vi "Lex String.vi"(8 "error in (no error)":errorcluster, 11 "JSON Lexer in":refnum<class "JSON Lexer.lvclass">) -> (0 "error out":errorcluster, 1 "EOF":bool, 2 "Next State":T1=enum."Value", 3 "JSON Lexer out":refnum<class "JSON Lexer.lvclass">)   [LabVIEW 2013, in "JKI JSON Serialization.lvlib" / "JSON Lexer.lvclass"]
uses:
  JSON Lexer.lvclass
  JSON Lexer States.ctl
  JSON Lexer.lvclass/JSON Lexer.ctl
  <vilib>/addons/_JKI.lib/Unicode/UTF-8 String/UTF-8 String.lvclass/UTF-8 String.ctl
  JSON Token Type.ctl
  <vilib>/addons/_JKI.lib/Unicode/UTF-8 String/Index Rune as UTF-8 Substring.vi
  <vilib>/addons/_JKI.lib/Unicode/UTF-8 String/Next Rune As UTF-8 Substring.vi
  <vilib>/addons/_JKI.lib/Unicode/UTF-8 String/Bytes In Rune.vi
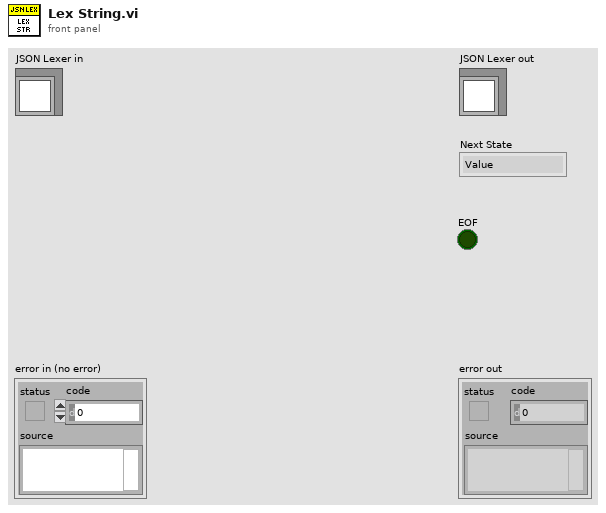
[diagram p1: front panel]
types:
  T1 = typedef "JKI JSON Serialization.lvlib/JSON Lexer.lvclass/JSON Lexer States.ctl" = enum16{"Undefined", "Value", "String", "Numeric", "Number", "Symbol", "Symbolic Number"}
  T2 = typedef "JKI JSON Serialization.lvlib/JSON Lexer.lvclass/JSON Token Type.ctl" = enum32{"unknown", "comma", "end-label", "begin-object", "end-object", "begin-array", "end-array", "quoted-string", "boolean", "exponential-number", "decimal-number", "integer-number", "special-number", "null", "symbol", "whitespace", "EOF"}
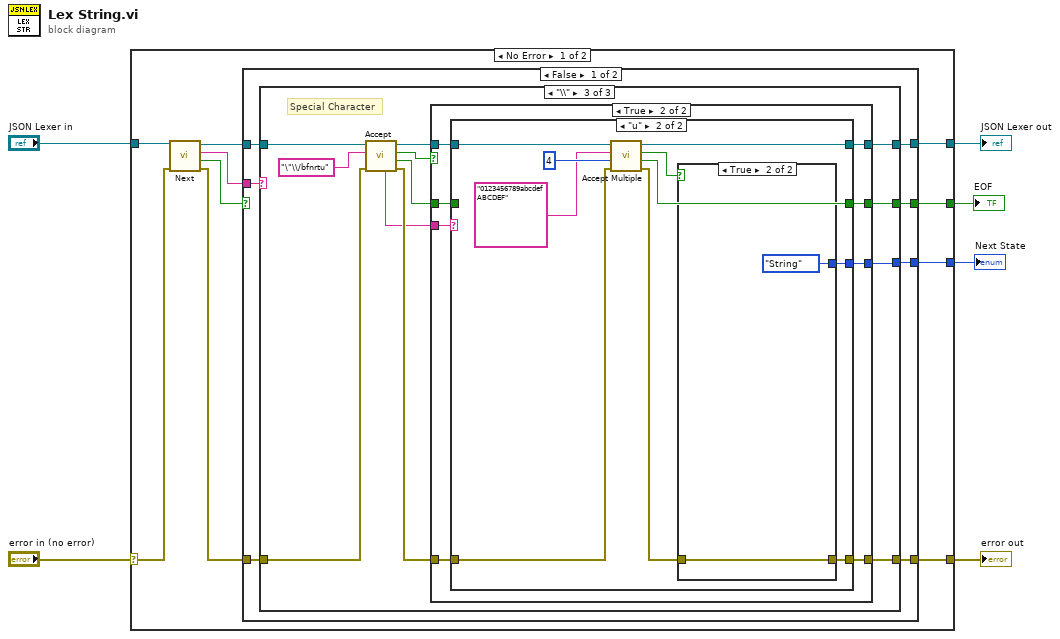
[diagram p0: block diagram]
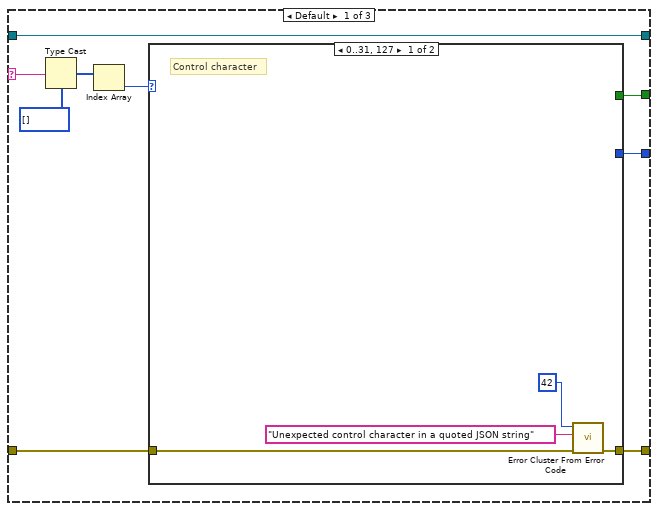
[diagram p2: hidden frame]
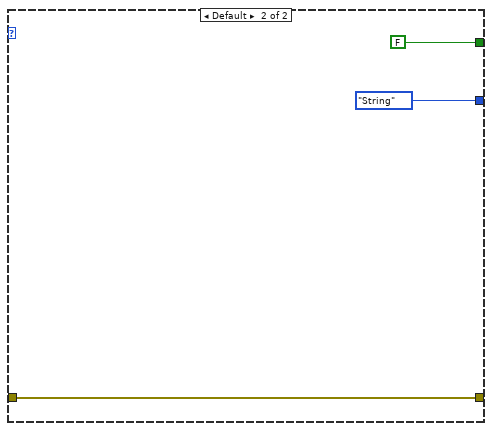
[diagram p3: hidden frame]
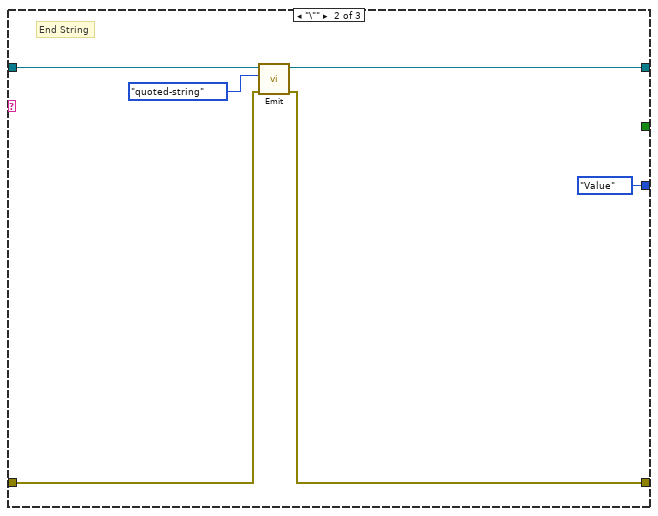
[diagram p4: hidden frame]
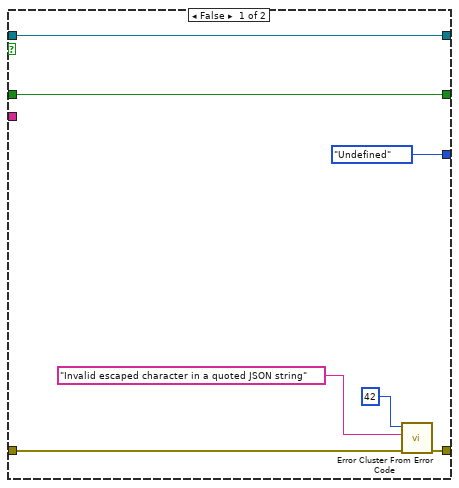
[diagram p5: hidden frame]
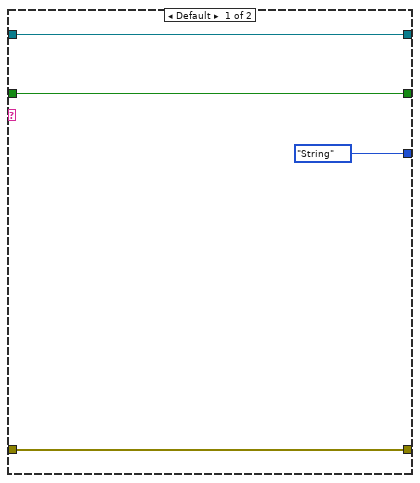
[diagram p6: hidden frame]
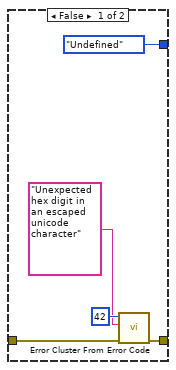
[diagram p7: hidden frame]
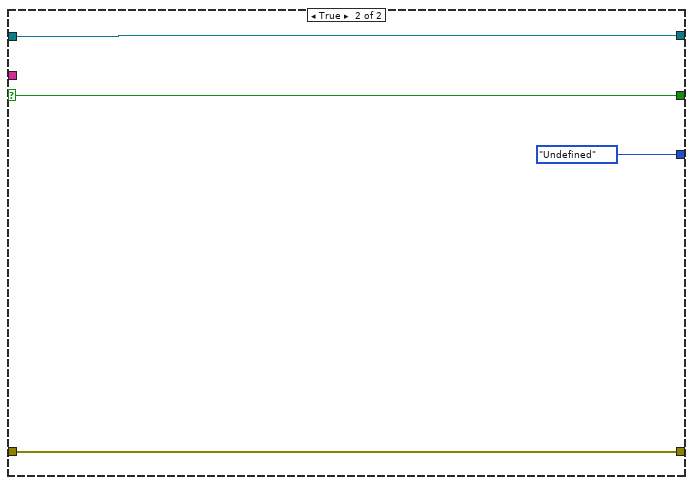
[diagram p8: hidden frame]
diagram:
  n1 = case shown="No Error" "error in (no error)" {
    selector: "error in (no error)" -> [w8 w99]
    tunnel: [w12 w99] -> w5
    tunnel: [w11 w98] -> w3
    tunnel: "JSON Lexer in" -> [w7 w98]
    tunnel: [w10 _] -> w2
    tunnel: [w9 _] -> w1
    frame No Error {
      n2 = call "Next.vi"("error in (no error)"=w8, "JSON Lexer in"=w7) -> ("error out"=w13:errorcluster, "EOF"=w16:bool, "Rune"=w15:string, "JSON Lexer out"=w14:refnum<class "JSON Lexer.lvclass">)  [unwired: 6 in]
      n3 = case shown="False" w16 {
        selector: w16 -> [_ w95]
        tunnel: w15 -> [w21 _]
        tunnel: w14 -> [w23 w97]
        tunnel: w13 -> [w20 w96]
        tunnel: [w19 w96] -> w12
        tunnel: [w22 w97] -> w11
        tunnel: [w18 w95] -> w10
        tunnel: [w17 JSON_Lexer_States."Undefined" ("Next State")] -> w9
        frame False {
          n4 = case shown="\"\\\\\"" w21 {
            selector: w21 -> [w29 _ _]
            tunnel: w23 -> [w32 w44 w57]
            tunnel: [w32 w43 w51] -> w22
            tunnel: w20 -> [w25 w42 w55]
            tunnel: [w24 w41 w50] -> w19
            tunnel: [w31 _ w49] -> w18
            tunnel: [w30 JSON_Lexer_States."Value" ("Next State") w47] -> w17
            frame Default {
              n5 = Type Cast(type=u8[] [], x=w29) -> (*(type *) &x=w27:u8[])
              n6 = Index Array(array=w27) -> (element=w26:u8)  [unwired: 1 in]
              n7 = case shown="0..31, 127" w26 {
                tunnel: [_ FALSE] -> w31
                tunnel: [_ JSON_Lexer_States."String" ("Next State")] -> w30
                tunnel: w25 -> [w35 w37]
                tunnel: [w36 w37] -> w24
                frame 0..31, 127 {
                  # "Control character"
                  n8 = call <vilib>:"Error Cluster From Error Code.vi"("error in (no error)"=w35, "error message (\"\")"="Unexpected control character in a quoted JSON string" ("error message (\"\")"), "error code (0)"=42) -> ("error out"=w36:errorcluster)  [unwired: 6 in]
                }
                frame Default {
                }
              }
            }
            frame "\"" {
              # "End String"
              n9 = call "Emit.vi"("error in (no error)"=w42, "JSON Token Type"=JSON_Token_Type."quoted-string", "JSON Lexer in"=w44) -> ("error out"=w41:errorcluster, "JSON Lexer out"=w43:refnum<class "JSON Lexer.lvclass">)  [unwired: 7 in]
            }
            frame "\\" {
              # "Special Character"
              n10 = call "Accept.vi"("error in (no error)"=w55, "Accepted Runes"="\"\\/bfnrtu", "JSON Lexer in"=w57) -> ("error out"=w54:errorcluster, "EOF"=w48:bool, "Accepted?"=w52:bool, "JSON Lexer out"=w53:refnum<class "JSON Lexer.lvclass">, "Rune"=w46:string)  [unwired: 4 in]
              n11 = case shown="True" w52 {
                tunnel: w54 -> [w61 w66]
                tunnel: w53 -> [w64 w71]
                tunnel: [w64 w70] -> w51
                tunnel: [w62 w65] -> w50
                tunnel: [w63 w69] -> w49
                tunnel: w48 -> [w63 w68]
                tunnel: [JSON_Lexer_States."Undefined" ("JSON Lexer State") w67] -> w47
                tunnel: w46 -> [_ w72]
                frame False {
                  n12 = call <vilib>:"Error Cluster From Error Code.vi"("error in (no error)"=w61, "error message (\"\")"="Invalid escaped character in a quoted JSON string" ("error message (\"\")"), "error code (0)"=42) -> ("error out"=w62:errorcluster)  [unwired: 6 in]
                }
                frame True {
                  n13 = case shown="\"u\"" w72 {
                    tunnel: w71 -> [w76 w86]
                    tunnel: [w76 w82] -> w70
                    tunnel: [w75 w78] -> w69
                    tunnel: w68 -> [w75 _]
                    tunnel: [JSON_Lexer_States."String" ("JSON Lexer State") w77] -> w67
                    tunnel: w66 -> [w73 w84]
                    tunnel: [w73 w81] -> w65
                    frame Default {
                    }
                    frame "u" {
                      n14 = call "Accept Multiple.vi"("error in (no error)"=w84, "Number"=4, "Accepted Runes"="0123456789abcdefABCDEF", "JSON Lexer in"=w86) -> ("error out"=w80:errorcluster, "EOF"=w78:bool, "Accepted?"=w79:bool, "JSON Lexer out"=w82:refnum<class "JSON Lexer.lvclass">)  [unwired: 4 in]
                      n15 = case shown="True" w79 {
                        tunnel: [w91 w93] -> w81
                        tunnel: w80 -> [w90 w93]
                        tunnel: [JSON_Lexer_States."Undefined" ("JSON Lexer State") JSON_Lexer_States."String" ("JSON Lexer State")] -> w77
                        frame False {
                          n16 = call <vilib>:"Error Cluster From Error Code.vi"("error in (no error)"=w90, "error message (\"\")"="Unexpected hex digit in an escaped unicode character" ("Accepted Runes"), "error code (0)"=42) -> ("error out"=w91:errorcluster)  [unwired: 6 in]
                        }
                        frame True {
                        }
                      }
                    }
                  }
                }
              }
            }
          }
        }
        frame True {
        }
      }
    }
    frame Error {
    }
  }
  "error out" <- w5
  "JSON Lexer out" <- w3
  "Next State" <- w1
  "EOF" <- w2
